vi "Contador.vi"() -> ()   [LabVIEW 2020]
panel:
  out "Boolean":bool
  in  "min":dbl
  in  "max":dbl
  in  "Referencia":dbl
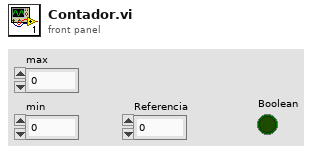
[diagram p1: front panel]
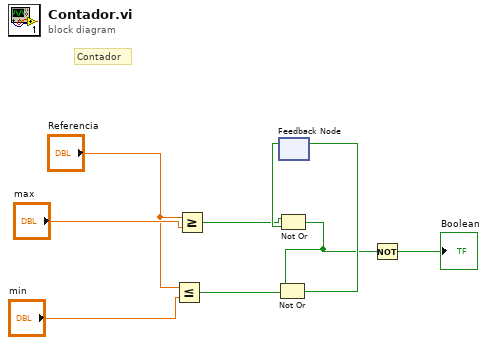
[diagram p0: block diagram]
diagram:
  # "Contador"
  n1 = Less Or Equal?(x="Referencia", y="min") -> (x <= y?=w7:bool)
  n2 = Greater Or Equal?(x="Referencia", y="max") -> (x >= y?=w1:bool)
  n3 = feedback #1() -> (w6:bool)  [unwired: 1 in]
  n4 = Not Or(1:w6, 2:w1) -> (0:w8:bool)
  n5 = Not Or(1:w7, 2:w8) -> (0:w9:bool)
  n6 = feedback-in #1(w9) -> ()
  n7 = Not(x=w8) -> (.not. x?=→"Boolean":bool)
